vi "WSVCAP SHL Host TL SPI Configure.vi"(9 "Clock Rate (Hz)":dbl=50000.0, 11 "error in":errorcluster, 13 "Log (T)":bool=TRUE) -> (6 "Actual Rate (Hz)":dbl, 15 "error out":errorcluster)   [LabVIEW 2012]
uses:
  Type Defs/WSVCAP SHL Function Enum.ctl
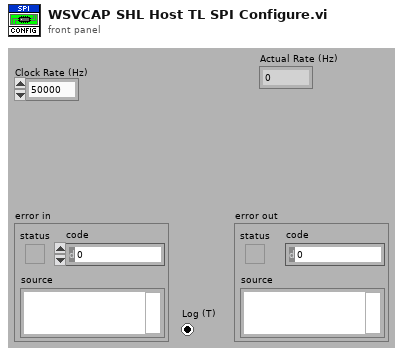
[diagram p1: front panel]
types:
  T1 = typedef "WSVCAP SHL Function Enum.ctl" = enum16{"Initialize", "Configure I2C", "Configure SPI", "Configure RFFE", "Write I2C", "Read I2C", "Write/Read SPI", "Start SPI Cycle", "Stop SPI Cycle", "Write RFFE", "Read RFFE", "Start RFFE Cycle", "Stop RFFE Cycle", "Get Status", "Close"}
  T2 = typedef "WSVCAP SHL Core System Cluster.ctl" = cluster{"Settings":T3, "FPGA Resource":tag, "Online":bool, "I2C Wait Ticks":u32, "SPI Wait Ticks":u32, "RFFE Wait Ticks":u32}
  T3 = typedef "WSVCAP SHL I2C Settings Cluster.ctl" = cluster{"FPGA Resource Name":string, "I2C Slave Address":u8, "I2C Clock Rate (Hz)":dbl, "SPI Clock Rate (Hz)":dbl, "RFFE Slave Address":u8, "RFFE Clock Rate (Hz)":dbl, "Simulate FPGA":bool, "C1 Cap DAC Default":u8, "C2 Cap DAC Default":u8, "C3 Cap DAC Default":u8}
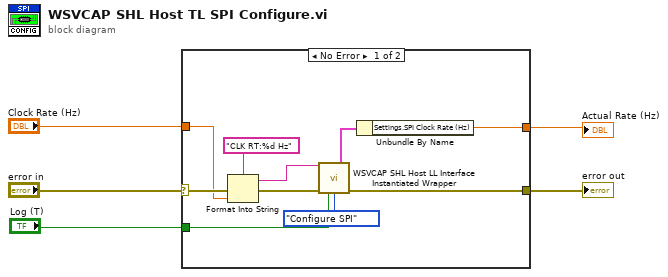
[diagram p0: block diagram]
diagram:
  n1 = case shown="No Error" "error in" {
    selector: "error in" -> [w11 w16]
    tunnel: [w15 w16] -> w5
    tunnel: [w13 _] -> w4
    tunnel: "Clock Rate (Hz)" -> [w9 _]
    tunnel: "Log (T)" -> [w6 _]
    frame No Error {
      n2 = Format Into String(format string="CLK RT:%d Hz", error in=w11, w9) -> (resulting string=w8:string, error out=w10:errorcluster)  [unwired: 1 in]
      n3 = call "WSVCAP SHL Host LL Interface Instantiated Wrapper.vi"("Message In"=w8, "error in"=w10, "Log (T)"=w6, "Function"=WSVCAP_SHL_Function_Enum."Configure SPI") -> ("System"=w14:T2, "error out"=w15:errorcluster)  [unwired: 9 in, 1 out]
      n4 = Unbundle By Name(w14) -> ("Settings.SPI Clock Rate (Hz)"=w13:dbl)
    }
    frame Error {
    }
  }
  "Actual Rate (Hz)" <- w4
  "error out" <- w5
